vi "DownloadInfo.vi"(8 "error in (no error)":errorcluster, 10 "hostname":string, 11 "USB download":path) -> (0 "error out":errorcluster)   [LabVIEW 2017, in "USBDrive.lvlib"]
uses:
  <vilib>/addons/InsightCM/Devices/Shared/Common/USBDrive/USBDrive.lvlib
  <vilib>/addons/InsightCM/Devices/Shared/Common/ServerComm/ServerComm.lvlib
  <vilib>/addons/SystemInfoProcess/SystemInfoProcess.lvlib
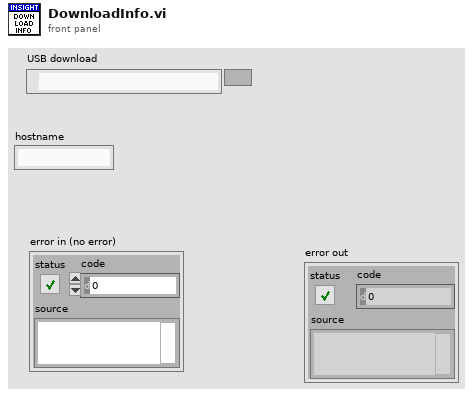
[diagram p1: front panel]
types:
  T1 = typedef "ConnectionInfo.ctl" = cluster{"ClientName":string, "TransceiverHost":string, "TransceiverPort":u16, "Password":string}
  T2 = typedef "SystemInfoProcess.lvlib/NetworkAdapterSettings.ctl" = cluster{"Adapter Mode":u32, "IsPrimary":bool, "MACAddr":string, "IP Address Request Mode":u32, "IPAddr":string, "SubnetMask":string, "Gateway":string, "DNSServer":string, "Alias":string}
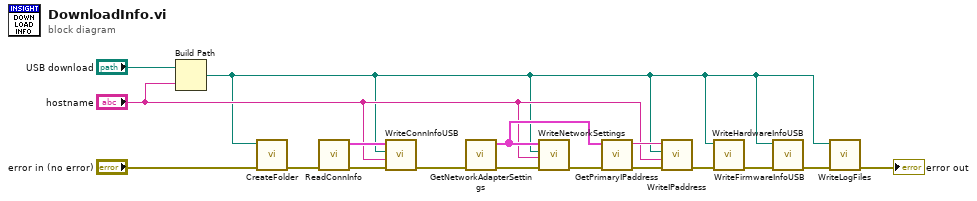
[diagram p0: block diagram]
diagram:
  n1 = Build Path(base path="USB download", name or relative path="hostname") -> (appended path=w3:path)
  n2 = call <vilib>:"CreateFolder.vi"("error in (no error)"="error in (no error)", "folder"=w3) -> ("error out"=w15:errorcluster)  [unwired: 8 in, 1 out]
  n3 = call <vilib>:"ReadConnInfo.vi"("error in (no error)"=w15) -> ("error out"=w16:errorcluster, "connection info"=w17:T1)  [unwired: 8 in, 1 out]
  n4 = call <vilib>:"WriteConnInfoUSB.vi"("error in (no error)"=w16, "hostname"="hostname", "path"=w3, "connection info"=w17) -> ("error out"=w14:errorcluster)  [unwired: 7 in]
  n5 = call <vilib>:"GetNetworkAdapterSettings.vi"("error in (no error)"=w14) -> ("error out"=w13:errorcluster, "Network Adapter Settings"=w10:T2[])  [unwired: 8 in, 1 out]
  n6 = call <vilib>:"WriteNetworkSettings.vi"("error in (no error)"=w13, "hostname"="hostname", "path"=w3, "network settings"=w10) -> ("error out"=w11:errorcluster)  [unwired: 7 in]
  n7 = call <vilib>:"GetPrimaryIPaddress.vi"("error in (no error)"=w11, "Network Adapter Settings"=w10) -> ("error out"=w9:errorcluster, "primary ip address"=w8:string)  [unwired: 8 in]
  n8 = call <vilib>:"WriteIPaddress.vi"("error in (no error)"=w9, "hostname"="hostname", "path"=w3, "ip address"=w8) -> ("error out"=w6:errorcluster)  [unwired: 7 in]
  n9 = call <vilib>:"WriteHardwareInfoUSB.vi"("error in (no error)"=w6, "path"=w3) -> ("error out"=w5:errorcluster)  [unwired: 9 in]
  n10 = call <vilib>:"WriteFirmwareInfoUSB.vi"("error in (no error)"=w5, "path"=w3) -> ("error out"=w4:errorcluster)  [unwired: 9 in]
  n11 = call <vilib>:"WriteLogFiles.vi"("error in (no error)"=w4, "path"=w3) -> ("error out"=→"error out":errorcluster)  [unwired: 9 in]
